vi "Configure Measurement.vi"(8 "error in (no error)":errorcluster, 9 "Enable Auto Range (F: Disable)":bool, 10 "Measurement Function (2: Current)":i32(ring)=2 items=["Off", "Volts", "Current", "Resistance"], 11 "VISA resource name":refnum<visa-resource-name>) -> (0 "error out":errorcluster, 3 "VISA resource name out":refnum<visa-resource-name>)   [LabVIEW 2017, in "ADCMT 6240.lvlib"]
doc: "Configures the measurement function and range on the instrument."
uses:
  ADCMT 6240.lvlib
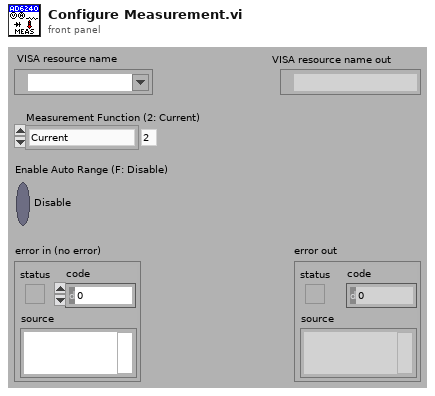
[diagram p1: front panel]
types:
  T1 = typedef "ADCMT 6240.lvlib/Extended User Data.ctl" = cluster{"Trigger Mode":u16, "Output Mode":u16, "Sample Count":i32, "Model":u16}
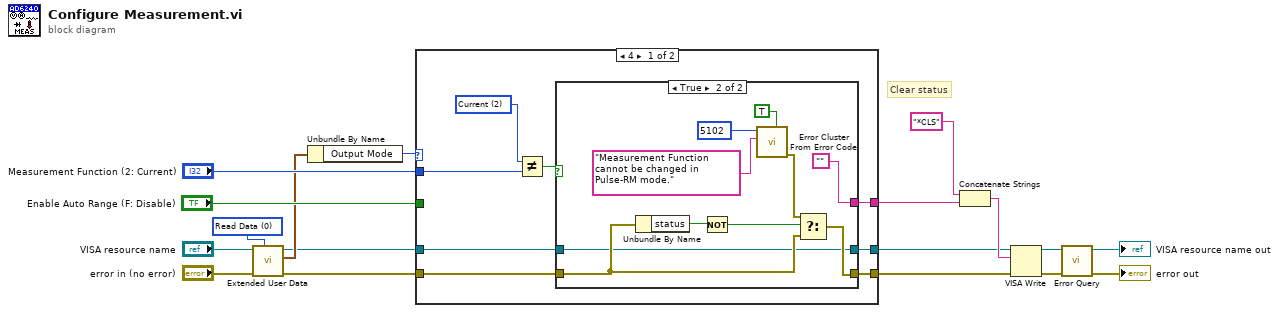
[diagram p0: block diagram]
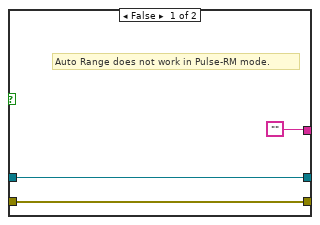
[diagram p2: hidden frame]
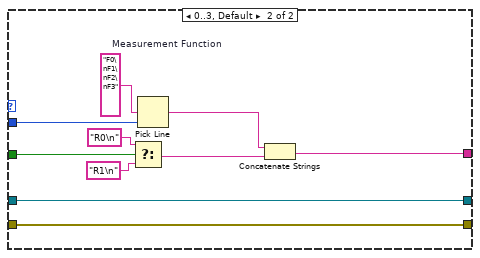
[diagram p3: hidden frame]
diagram:
  w10 = u16 0 items=["Read Data", "Write Data", "Dispose of Data"] ("Action")
  # "Clear status"
  n1 = call "Extended User Data.vi"("Action"=w10, "Error In (no error)"="error in (no error)", "VISA resource name in"="VISA resource name") -> ("Error Out"=w5:errorcluster, "User Data Out"=w7:T1, "VISA resource name out"=w3:refnum<visa-resource-name>)  [unwired: 6 in]
  n2 = Unbundle By Name(w7) -> ("Output Mode"=w6:u16)
  n3 = case shown="4" w6 {
    tunnel: "Measurement Function (2: Current)" -> [w23 w49]
    tunnel: "Enable Auto Range (F: Disable)" -> [_ w46]
    tunnel: [w26 w42] -> w1
    tunnel: w5 -> [w24 w44]
    tunnel: [w25 w44] -> w4
    tunnel: w3 -> [w20 w43]
    tunnel: [w19 w43] -> w2
    frame 4 {
      w22 = u16 2 items=["Off", "Volts", "Current", "Resistance"] ("Measurement Function (2: Current)")
      n4 = Not Equal?(x=w22, y=w23) -> (x != y?=w21:bool)
      n5 = case shown="True" w21 {
        tunnel: ["" ""] -> w26
        tunnel: [w29 w34] -> w25
        tunnel: w24 -> [w29 w33]
        tunnel: w20 -> [w28 w31]
        tunnel: [w28 w31] -> w19
        frame False {
          # "Auto Range does not work in Pulse-RM mode."
        }
        frame True {
          n6 = Unbundle By Name(w33) -> ("status"=w36:bool)
          n7 = Not(x=w36) -> (.not. x?=w35:bool)
          n8 = call <vilib>:"Error Cluster From Error Code.vi"("is warning? (False)"=TRUE ("show call chain? (False)"), "error message (\"\")"="Measurement Function  cannot be changed in Pulse-RM mode." ("Source (VI Name)"), "error code (0)"=5102 ("Code")) -> ("error out"=w32:errorcluster)  [unwired: 6 in]
          n9 = Select(t=w32, s=w35, f=w33) -> (s? t:f=w34:errorcluster)
        }
      }
    }
    frame 0..3, Default {
      w45 = "F0\nF1\nF2\nF3"  # Measurement Function
      n10 = Select(t="R0\n", s=w46, f="R1\n") -> (s? t:f=w41:string)
      n11 = Pick Line(multi-line string=w45, line index=w49) -> (output string=w40:string)  [unwired: 1 in]
      n12 = Concatenate Strings(w40, w41) -> (w42:string)
    }
  }
  n13 = Concatenate Strings("*CLS", w1) -> (w12:string)
  n14 = VISA Write(VISA resource name=w2, write buffer=w12, error in (no error)=w4) -> (VISA resource name out=w15:refnum<visa-resource-name>, error out=w14:errorcluster)  [unwired: 1 out]
  n15 = call "Error Query.vi"("error in (no error)"=w14, "VISA resource name"=w15) -> ("error out"=→"error out":errorcluster, "VISA resource name out"=→"VISA resource name out":refnum<visa-resource-name>)  [unwired: 6 in, 2 out]
